vi "DAQ_Voltage.vi"() -> ()   [LabVIEW 2020]
panel:
  in  "file path (use dialog)":path
  in  "number of samples":i32=100
  out "Waveform Chart":dynamicdata(graph)
  in  "stop (F)":bool
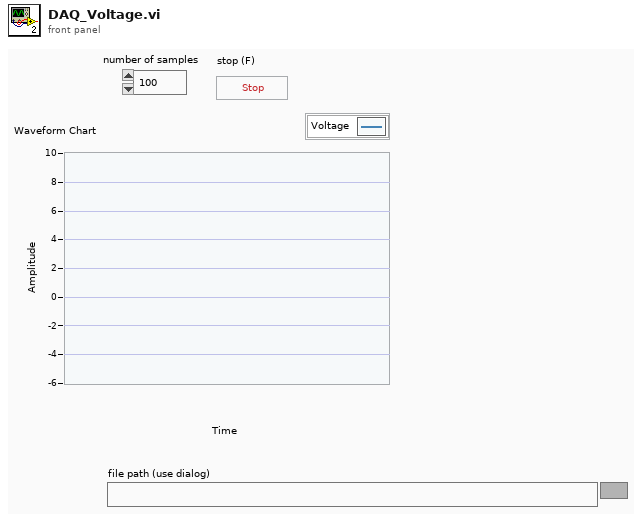
[diagram p1: front panel]
types:
  T1 = enum16{"open", "replace", "create", "open or create", "replace or create", "replace or create with confirmation"}
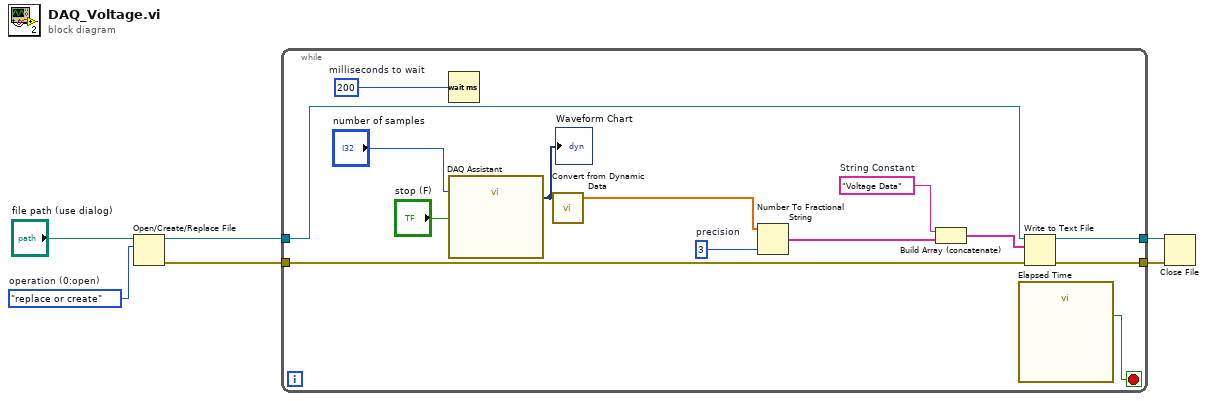
[diagram p0: block diagram]
diagram:
  w5 = T1."replace or create"  # operation (0:open)
  n1 = Open/Create/Replace File(file path (use dialog)="file path (use dialog)", operation (0:open)=w5) -> (refnum out=w4:refnum<file>, error out=w3:errorcluster)  [unwired: 4 in, 1 out]
  n2 = while {
    tunnel: w4 -> [w17]
    tunnel: w3 -> [w16]
    tunnel: [w15] -> w2
    tunnel: [w14] -> w1
    stop <- w18 stop-if-true
    w7 = u32 200  # milliseconds to wait
    w11 = "Voltage Data"  # String Constant
    w10 = i16 3  # precision
    n3 = Wait (ms)(milliseconds to wait=w7) -> ()  [unwired: 1 out]
    n4 = call "DAQ Assistant"("number of samples"="number of samples", "stop (F)"="stop (F)") -> ("data"=w13:dynamicdata)  [unwired: 14 in, 3 out]
    "Waveform Chart" <- w13
    n5 = call "Convert from Dynamic Data"("Dynamic Data Type"=w13) -> ("Array"=w9:dbl[])  [unwired: 3 in]
    n6 = Number To Fractional String(number=w9, precision (6)=w10) -> (F-format string=w12:string[])  [unwired: 2 in]
    n7 = Build Array (concatenate) "Build Array"(w11, w12) -> (w8:string[])
    n8 = call "Elapsed Time"() -> ("Time has Elapsed"=w18:bool)  [unwired: 12 in, 7 out]
    n9 = Write to Text File(file (use dialog)=w17, text=w8, error in=w16) -> (refnum out=w15:refnum<file>, error out=w14:errorcluster)  [unwired: 1 in, 1 out]
  }
  n10 = Close File(refnum=w2, error in=w1) -> ()  [unwired: 2 out]
